vi "macro_ProfiledPIDController_Execute.vi"   [LabVIEW 2019, in "Trajectory_Library.lvlib"]
uses:
  Trajectory_Library.lvlib
types:
  T1 = typedef "Trajectory_Library.lvlib/PID_TUNING.ctl" = cluster{"Kp":dbl, "Ki":dbl, "Kd":dbl, "MaximumIntegral":dbl, "MinimumIntegral":dbl}
  T2 = typedef "WPILib_Math.lvlib/PID_INPUT_LIMITS.ctl" = cluster{"MaxInput":dbl, "MinInput":dbl, "Continuous":bool}
  T3 = typedef "WPILib_Math.lvlib/TRAPEZOID_PROFILE_CONSTRAINT.ctl" = cluster{"MaxVelocity":dbl, "MaxAcceleration":dbl}
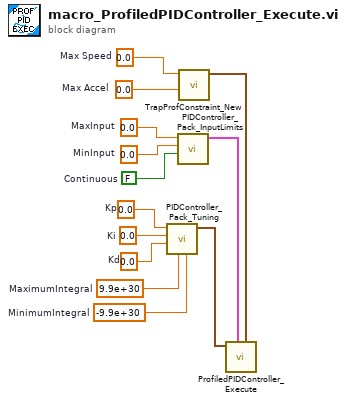
[diagram p0: block diagram]
diagram:
  w1 = 0.0  # Max Speed
  w2 = 0.0  # Max Accel
  w4 = 0.0  # MaxInput
  w5 = 0.0  # MinInput
  w6 = FALSE  # Continuous
  w7 = 0.0  # Kp
  w8 = 0.0  # Ki
  w9 = 0.0  # Kd
  w10 = 9.9e+30  # MaximumIntegral
  w11 = -9.9e+30  # MinimumIntegral
  n1 = call "PIDController_Pack_Tuning.vi"("MinimumIntegral"=w11, "MaximumIntegral"=w10, "Kd"=w9, "Ki"=w8, "Kp"=w7) -> ("PID Tuning"=w12:T1)  [unwired: 6 in]
  n2 = call "PIDController_Pack_InputLimits.vi"("Continuous"=w6, "MinInput"=w5, "MaxInput"=w4) -> ("PID Input Limits"=w13:T2)  [unwired: 8 in]
  n3 = call "TrapProfConstraint_New.vi"("Max Accel"=w2, "Max Speed (M/S)"=w1) -> ("TRAPEZOID_PROFILE_CONSTRAINT"=w3:T3)  [unwired: 9 in]
  n4 = call "ProfiledPIDController_Execute.vi"("Constraints"=w3, "PID Input Limits"=w13, "PID Tuning"=w12) -> ()  [unwired: 5 in, 4 out]
